vi "dBtoRI.vi"(10 "Phase":dbl[][](array[numeric]), 11 "dB":dbl[][](array[numeric])) -> (2 "b":dbl[][](array[numeric]), 3 "a":dbl[][](array[numeric]))   [LabVIEW 2011]
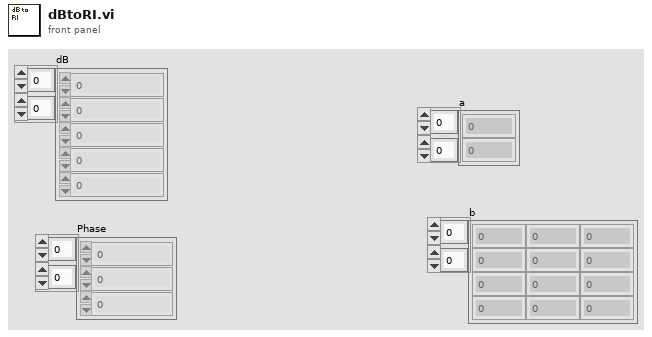
[diagram p1: front panel]
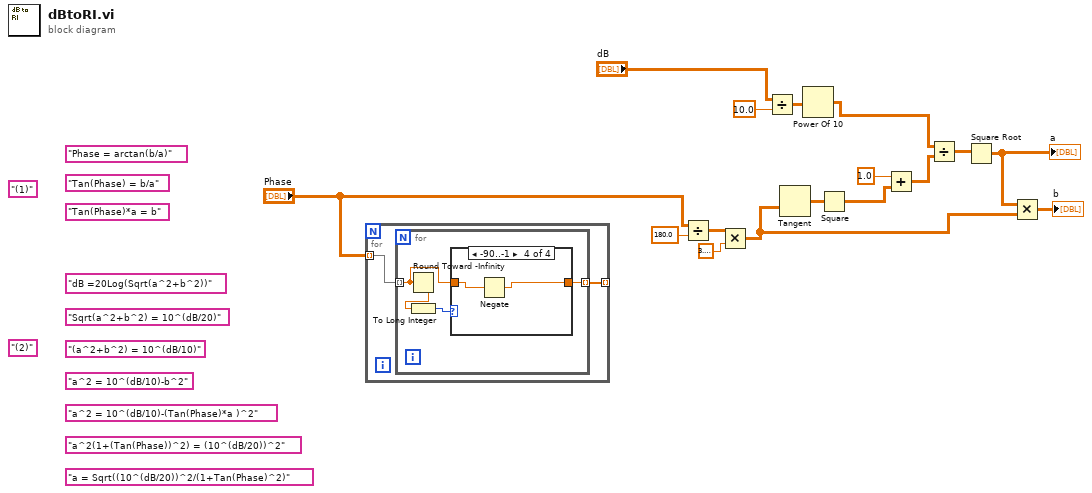
[diagram p0: block diagram]
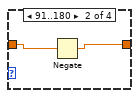
[diagram p3: hidden frame]
diagram:
  (unwired) "(2)"
  (unwired) "(1)"
  (unwired) "a = Sqrt((10^(dB/20))^2/(1+Tan(Phase)^2)"
  (unwired) "a^2(1+(Tan(Phase))^2) = (10^(dB/20))^2"
  (unwired) "a^2 = 10^(dB/10)-(Tan(Phase)*a )^2"
  (unwired) "Tan(Phase)*a = b"
  (unwired) "a^2 = 10^(dB/10)-b^2"
  (unwired) "(a^2+b^2) = 10^(dB/10)"
  (unwired) "Sqrt(a^2+b^2) = 10^(dB/20)"
  (unwired) "Tan(Phase) = b/a"
  (unwired) "dB =20Log(Sqrt(a^2+b^2))"
  (unwired) "Phase = arctan(b/a)"
  n1 = for {
    tunnel: "Phase" -> [w18] mode=indexing
    tunnel: [w17] -> _ mode=indexing
    n2 = for {
      tunnel: w18 -> [w20] mode=indexing
      tunnel: [w19] -> w17 mode=indexing
      n3 = Round Toward -Infinity(1:w20) -> (0:w22:dbl)
      n4 = To Long Integer(number=w22) -> (32bit integer=w21:i32)
      n5 = case shown="-90..-1" w21 {
        tunnel: w20 -> [w23 w25 w26 w28]
        tunnel: [w23 w24 w26 w27] -> w19
        frame 0..90, Default {
        }
        frame 91..180 {
          n6 = Negate(x=w25) -> (-x=w24:dbl)
        }
        frame -180..-91 {
        }
        frame -90..-1 {
          n7 = Negate(x=w28) -> (-x=w27:dbl)
        }
      }
    }
  }
  n8 = Divide(x="Phase", y=180.0) -> (x/y=w4:dbl[][])
  n9 = Multiply(x=w4, y=3.141592653589793) -> (x*y=w2:dbl[][])
  n10 = Divide(x="dB", y=10.0) -> (x/y=w14:dbl[][])
  n11 = Tangent(1:w2) -> (0:w7:dbl[][])
  n12 = Power Of 10(x=w14) -> (10^x=w8:dbl[][])
  n13 = Square(x=w7) -> (x^2=w6:dbl[][])
  n14 = Add(x=1.0, y=w6) -> (x+y=w12:dbl[][])
  n15 = Divide(x=w8, y=w12) -> (x/y=w11:dbl[][])
  n16 = Square Root(x=w11) -> (sqrt(x)=w10:dbl[][])
  "a" <- w10
  n17 = Multiply(x=w10, y=w2) -> (x*y=→"b":dbl[][])
